vi "Laser Engraver.vi"() -> ()   [LabVIEW 2023]
uses:
  <vilib>/addons/database/Connection.llb/DB Tools Open Connec (String).vi
  <vilib>/regexp/Match Regular Expression.xnode
  <vilib>/addons/database/NI_Database_API.lvlib
panel:
  out "Full Work Order":string caption="Work Order"
  out "Quantity":string
  out "Subnumber":string caption="Work Order"
  out "System Status":string
  in  "Laser Etcher":refnum<visa-resource-name>
  out "Status":string
  out "error out":errorcluster
  in  "stop":bool
  in  "Start":bool
  out "Work Order":string
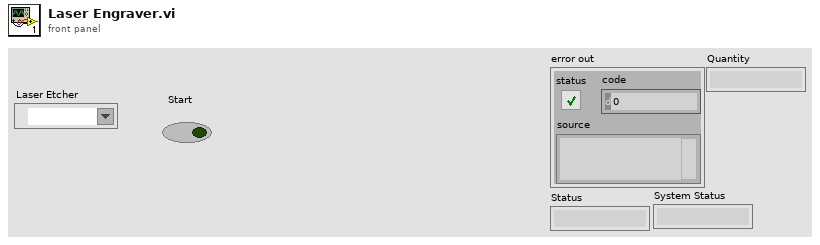
[diagram p1: front panel]
types:
  T1 = typedef "NI_Database_API.lvlib/Conn ObjectReference.ctl" = refnum<k1>
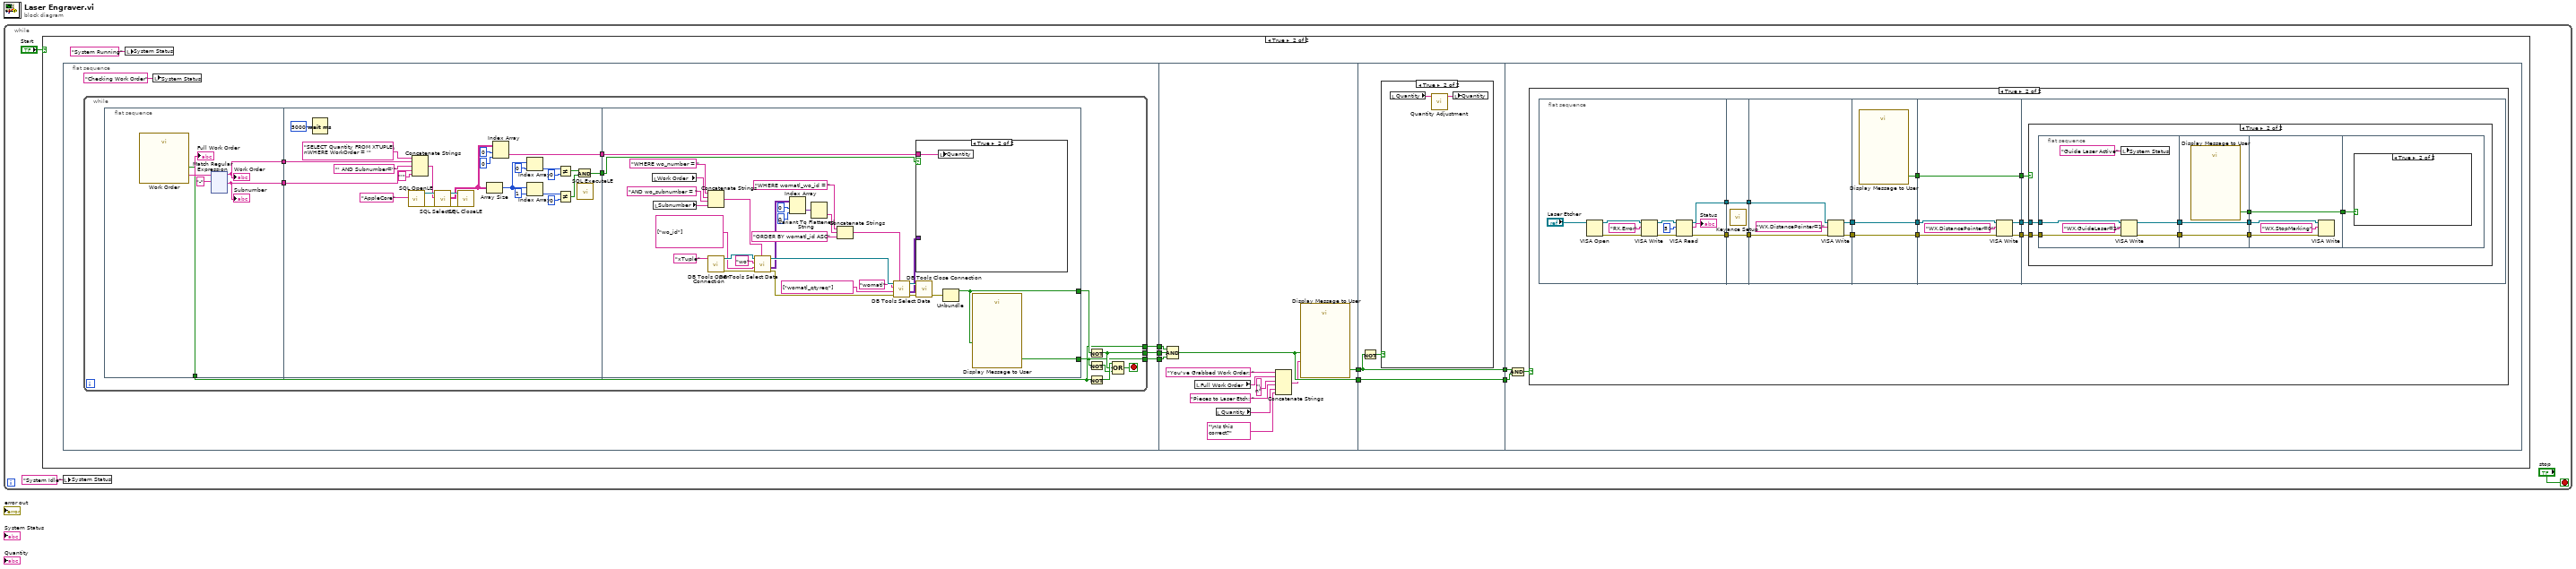
[diagram p0: block diagram]
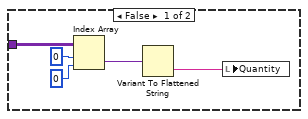
[diagram p3: hidden frame]
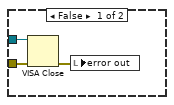
[diagram p6: hidden frame]
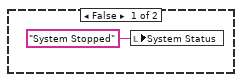
[diagram p7: hidden frame]
diagram:
  n1 = while {
    stop <- "stop" stop-if-true
    n2 = case shown="True" "Start" {
      frame False {
      }
      frame True {
        n3 = flat-sequence {
          tunnel: [w14] -> w10
          tunnel: [w15] -> w9
          tunnel: [w13] -> w8
          tunnel: w10 -> [w222]
          tunnel: w9 -> [w221]
          tunnel: w8 -> [w220]
          tunnel: [w219] -> w7
          tunnel: [w218] -> w5
          tunnel: w7 -> [w224]
          tunnel: [w224] -> w6
          tunnel: w5 -> [w225]
          tunnel: [w225] -> w4
          tunnel: w6 -> [w230]
          tunnel: w4 -> [w229]
          frame #0 {
            n4 = while {
              tunnel: [w23] -> w15
              tunnel: [w21] -> w14
              tunnel: [w20] -> w13
              stop <- w25 stop-if-true
              n5 = flat-sequence {
                tunnel: [w29] -> w21
                tunnel: [w28] -> w18
                tunnel: [w27] -> w17
                tunnel: [w159] -> w19
                tunnel: w18 -> [w155]
                tunnel: w17 -> [w154]
                tunnel: [w149] -> w16
                tunnel: [w178] -> w26
                tunnel: [w192] -> w20
                tunnel: w19 -> [w177]
                tunnel: w16 -> [w176]
                frame #0 {
                  n6 = call "Work Order"() -> ("Work Order"=w31:string, "OK"=w29:bool)  [unwired: 17 in, 1 out]
                  "Full Work Order" <- w31
                  n7 = xnode "Match Regular Expression"("input string"=w31, "regular expression"="-") -> ("before match"=w27:string, "after match"=w28:string)  [unwired: 4 in, 3 out]
                  "Work Order" <- w27
                  "Subnumber" <- w28
                }
                frame #1 {
                  n8 = Wait (ms)(milliseconds to wait=u32 5000) -> ()  [unwired: 1 out]
                  n9 = call "SQL OpenLE.vi"("ConnectionString In"="AppleCore") -> ("Connection Out"=w173:refnum<k7>, "Error out"=w172:errorcluster)  [unwired: 17 in]
                  n10 = Concatenate Strings("SELECT Quantity FROM XTUPLE\nWHERE WorkOrder = '" ("SQL Query"), w154, "' AND Subnumber='" ("string"), w155, "'" ("string")) -> (w153:string)
                  n11 = call "SQL SelectLE.vi"("Connection In"=w173, "SQL Query"=w153, "Error in (no error)"=w172) -> ("Connection Out"=w170:refnum<k7>, "Data"=w152:string[][], "Error out"=w169:errorcluster)  [unwired: 14 in]
                  n12 = call "SQL CloseLE.vi"("Connection In"=w170, "Error in (no error)"=w169) -> ()  [unwired: 17 in, 1 out]
                  n13 = Array Size(array=w152) -> (size(s)=w168:i32[])
                  n14 = Index Array(array=w152, index (row)=0, index (col)=0 ("disabled index (col)")) -> (element=w149:string)
                  n15 = Index Array(array=w168, index=0) -> (element=w163:i32)
                  n16 = Index Array(array=w168, index=1) -> (element=w165:i32)
                  n17 = Not Equal?(x=w163, y=0) -> (x != y?=w161:bool)
                  n18 = Not Equal?(x=w165, y=0) -> (x != y?=w160:bool)
                  n19 = And(x=w161, y=w160) -> (x .and. y?=w159:bool)
                  n20 = call "SQL ExecuteLE.vi"() -> ()  [unwired: 18 in, 2 out]
                }
                frame #2 {
                  n21 = local read "Work Order"() -> (w201:string)
                  n22 = local read "Subnumber"() -> (w175:string)
                  n23 = Concatenate Strings("WHERE wo_number = " ("condition"), w201, "AND wo_subnumber = " ("string"), w175) -> (w202:string)
                  n24 = call-poly <vilib>:"DB Tools Open Connection.vi"("connection information"="xTuple" ("Connection Strings")) -> ("error out"=w199:errorcluster, "connection reference"=w200:T1)  [unwired: 7 in]
                  n25 = call <vilib>:"DB Tools Select Data.vi"("condition"=w202, "error in (no error)"=w199, "columns"=string[] ["wo_id"], "table"="wo", "connection reference"=w200) -> ("error out"=w204:errorcluster, "data"=w188:variant[][], "connection reference out"=w203:T1)  [unwired: 1 in]
                  n26 = Index Array(array=w188, index (row)=0, index (col)=0 ("disabled index (col)")) -> (element=w184:variant)
                  n27 = Variant To Flattened String(Variant=w184) -> (data string=w183:string)  [unwired: 1 out]
                  n28 = Concatenate Strings("WHERE womatl_wo_id = " ("condition"), w183, "ORDER BY womatl_id ASC" ("string")) -> (w181:string)
                  n29 = call <vilib>:"DB Tools Select Data.vi"("condition"=w181, "error in (no error)"=w204, "columns"=string[] ["womatl_qtyreq"], "table"="womatl", "connection reference"=w203) -> ("error out"=w190:errorcluster, "data"=w179:variant[][], "connection reference out"=w191:T1)  [unwired: 1 in]
                  n30 = case shown="True" w177 {
                    tunnel: w179 -> [w207 _]
                    tunnel: w176 -> [_ w210]
                    frame False {
                      n31 = Index Array(array=w207, index (row)=0, index (col)=0) -> (element=w206:variant)
                      n32 = Variant To Flattened String(Variant=w206) -> (data string=w205:string)  [unwired: 1 out]
                      n33 = local write "Quantity"(w205) -> ()
                    }
                    frame True {
                      n34 = local write "Quantity"(w210) -> ()
                    }
                  }
                  n35 = call <vilib>:"DB Tools Close Connection.vi"("error in (no error)"=w190, "connection reference"=w191) -> ("error out"=w193:errorcluster)  [unwired: 5 in]
                  n36 = Unbundle(w193) -> ("status"=w178:bool)  [unwired: 2 out]
                  n37 = call "Display Message to User"("Enable"=w178) -> ("OK"=w192:bool)  [unwired: 9 in, 1 out]
                }
              }
              n38 = Not(x=w26) -> (.not. x?=w23:bool)
              n39 = Not(x=w20) -> (.not. x?=w22:bool)
              n40 = Not(x=w21) -> (.not. x?=w24:bool)
              n41 = Compound Arithmetic op=OR(w24, w23, w22) -> (w25:bool)
            }
            n42 = local write "System Status"("Checking Work Order" ("System Status")) -> ()
          }
          frame #1 {
            n43 = Compound Arithmetic op=AND(w222, w221, w220) -> (w218:bool)
            n44 = local read "Full Work Order"() -> (w216:string)
            n45 = local read "Quantity"() -> (w212:string)
            n46 = Concatenate Strings("You've Grabbed Work Order: " ("Message"), w216, "\n" ("string"), "Pieces to Laser Etch: " ("string"), w212, "\nIs this correct?" ("string")) -> (w213:string)
            n47 = call "Display Message to User"("Enable"=w218, "Message"=w213) -> ("Yes"=w219:bool)  [unwired: 8 in, 1 out]
          }
          frame #2 {
            n48 = Not(x=w224) -> (.not. x?=w223:bool)
            n49 = case shown="True" w223 {
              frame False {
              }
              frame True {
                n50 = local read "Quantity"() -> (w227:string)
                n51 = call "Quantity Adjustment.vi"("Quantity"=w227) -> ("Quantity (Updated)"=w226:string)  [unwired: 10 in]
                n52 = local write "Quantity"(w226) -> ()
              }
            }
          }
          frame #3 {
            n53 = Compound Arithmetic op=AND(w230, w229) -> (w228:bool)
            n54 = case shown="True" w228 {
              frame False {
              }
              frame True {
                n55 = flat-sequence {
                  tunnel: [w245] -> w234
                  tunnel: [w244] -> w232
                  tunnel: w234 -> [w254]
                  tunnel: [w254] -> w233
                  tunnel: w232 -> [w253]
                  tunnel: [w253] -> w231
                  tunnel: [w258] -> w242
                  tunnel: w233 -> [w255]
                  tunnel: [w257] -> w241
                  tunnel: w231 -> [w256]
                  tunnel: w242 -> [w262]
                  tunnel: [w262] -> w240
                  tunnel: w241 -> [w261]
                  tunnel: [w261] -> w239
                  tunnel: [w260] -> w238
                  tunnel: w240 -> [w264]
                  tunnel: [w266] -> w237
                  tunnel: w239 -> [w263]
                  tunnel: [w265] -> w236
                  tunnel: [w267] -> w235
                  tunnel: w238 -> [w267]
                  tunnel: w237 -> [w271]
                  tunnel: w236 -> [w270]
                  tunnel: w235 -> [w269]
                  frame #0 {
                    n56 = VISA Open(VISA resource name="Laser Etcher") -> (VISA resource name=w247:refnum<visa-resource-name>, error out=w250:errorcluster)  [unwired: 4 in]
                    n57 = VISA Write(VISA resource name=w247, write buffer="RX,Error", error in (no error)=w250) -> (VISA resource name out=w248:refnum<visa-resource-name>, error out=w249:errorcluster)  [unwired: 1 out]
                    n58 = VISA Read(VISA resource name=w248, byte count=u32 5, error in (no error)=w249) -> (VISA resource name out=w245:refnum<visa-resource-name>, read buffer=→"Status":string, error out=w244:errorcluster)  [unwired: 1 out]
                  }
                  frame #1 {
                    n59 = call "Keyance Setup.vi"() -> ()  [unwired: 10 in, 2 out]
                  }
                  frame #2 {
                    n60 = VISA Write(VISA resource name=w255, write buffer="WX,DistancePointer=1", error in (no error)=w256) -> (VISA resource name out=w258:refnum<visa-resource-name>, error out=w257:errorcluster)  [unwired: 1 out]
                  }
                  frame #3 {
                    n61 = call "Display Message to User"() -> ("OK"=w260:bool)  [unwired: 10 in, 1 out]
                  }
                  frame #4 {
                    n62 = VISA Write(VISA resource name=w264, write buffer="WX,DistancePointer=0", error in (no error)=w263) -> (VISA resource name out=w266:refnum<visa-resource-name>, error out=w265:errorcluster)  [unwired: 1 out]
                  }
                  frame #5 {
                    n63 = case shown="True" w269 {
                      tunnel: w270 -> [w273 w276]
                      tunnel: w271 -> [w274 w275]
                      frame False {
                        n64 = VISA Close(VISA resource name=w274, error in (no error)=w273) -> (error out=w272:errorcluster)
                        n65 = local write "error out"(w272) -> ()
                      }
                      frame True {
                        n66 = flat-sequence {
                          tunnel: [w286] -> w282
                          tunnel: [w285] -> w281
                          tunnel: w276 -> [w284]
                          tunnel: w275 -> [w283]
                          tunnel: [w291] -> w280
                          tunnel: [w290] -> w279
                          tunnel: w282 -> [w290]
                          tunnel: [w289] -> w278
                          tunnel: w281 -> [w289]
                          tunnel: [w294] -> w277
                          tunnel: w280 -> [w294]
                          tunnel: w279 -> [w293]
                          tunnel: w278 -> [w292]
                          tunnel: w277 -> [w296]
                          frame #0 {
                            n67 = local write "System Status"("Guide Laser Active" ("System Status")) -> ()
                            n68 = VISA Write(VISA resource name=w283, write buffer="WX,GuideLaser=2", error in (no error)=w284) -> (VISA resource name out=w286:refnum<visa-resource-name>, error out=w285:errorcluster)  [unwired: 1 out]
                          }
                          frame #1 {
                            n69 = call "Display Message to User"() -> ("OK"=w291:bool)  [unwired: 10 in, 1 out]
                          }
                          frame #2 {
                            n70 = VISA Write(VISA resource name=w293, write buffer="WX,StopMarking", error in (no error)=w292) -> ()  [unwired: 3 out]
                          }
                          frame #3 {
                            n71 = case shown="True" w296 {
                              frame False {
                                n72 = local write "System Status"("System Stopped" ("System Status")) -> ()
                              }
                              frame True {
                              }
                            }
                          }
                        }
                      }
                    }
                  }
                }
              }
            }
          }
        }
        n73 = local write "System Status"("System Running") -> ()
      }
    }
    n74 = local write "System Status"("System Idle") -> ()
  }
